vi "subFiniteRx.vi"(0 "IVI Refnum in":refnum<k15>, 1 "Active Antenna":string(combo)="RX2", 5 "Number of Samples":i32, 9 "Carrier Frequency":dbl, 11 "error in (no error)":errorcluster) -> (4 "IVI Refnum out":refnum<k15>, 6 "data":cdb[](array[numeric]), 15 "error out":errorcluster)   [LabVIEW 2011]
uses:
  <instrlib>/niUSRP/niUSRP Fetch Rx Data (CDB).vi
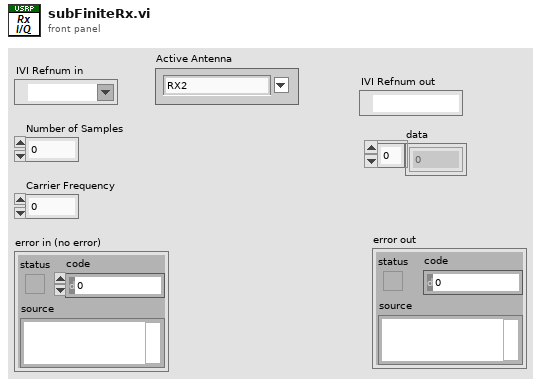
[diagram p1: front panel]
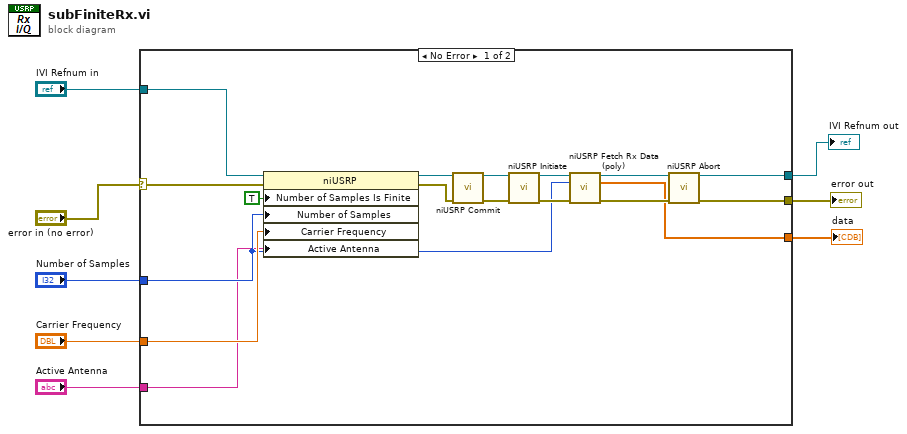
[diagram p0: block diagram]
diagram:
  n1 = case shown="No Error" "error in (no error)" {
    selector: "error in (no error)" -> [w9 w27]
    tunnel: [w24 w27] -> w8
    tunnel: [w23 w26] -> w7
    tunnel: "Carrier Frequency" -> [w21 _]
    tunnel: "IVI Refnum in" -> [w17 w26]
    tunnel: "Number of Samples" -> [w16 _]
    tunnel: [w11 _] -> w3
    tunnel: "Active Antenna" -> [w10 _]
    frame No Error {
      n2 = property class="niUSRP"(reference=w17, error in=w9, "Number of Samples Is Finite"=TRUE ("Configuration:Number of Samples Is Finite"), "Number of Samples"=w16, "Carrier Frequency"=w21, "Active Antenna"=w10) -> (reference out=w15:refnum<k15>, error out=w14:errorcluster)
      n3 = call <instrlib>:"niUSRP Commit.vi"("session handle"=w15, "error in (no error)"=w14) -> ("session handle out"=w13:refnum<k15>, "error out"=w12:errorcluster)  [unwired: 12 in]
      n4 = call <instrlib>:"niUSRP Initiate.vi"("session handle"=w13, "error in (no error)"=w12) -> ("session handle out"=w19:refnum<k15>, "error out"=w20:errorcluster)  [unwired: 12 in]
      n5 = call-poly <instrlib>:"niUSRP Fetch Rx Data (poly).vi"("session handle"=w19, "number of samples"=w16, "error in (no error)"=w20) -> ("session handle out"=w22:refnum<k15>, "data"=w11:cdb[], "error out"=w25:errorcluster)  [unwired: 9 in, 1 out]
      n6 = call <instrlib>:"niUSRP Abort.vi"("session handle"=w22, "error in (no error)"=w25) -> ("session handle out"=w23:refnum<k15>, "error out"=w24:errorcluster)  [unwired: 12 in]
    }
    frame Error {
    }
  }
  "data" <- w3
  "error out" <- w8
  "IVI Refnum out" <- w7
